vi "Single Beep.vi"(0 "Number of Tones (Def=1)":i32=1) -> ()   [LabVIEW 2020]
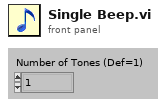
[diagram p1: front panel]
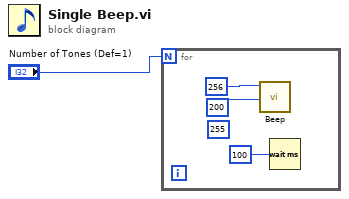
[diagram p0: block diagram]
diagram:
  n1 = for {
    N: "Number of Tones (Def=1)" -> [_]
    (unwired) 255
    n2 = call <vilib>:"Beep.vi"("duration (msec)"=200, "frequency (Hz)"=256) -> ()  [unwired: 10 in]
    n3 = Wait (ms)(milliseconds to wait=100) -> ()  [unwired: 1 out]
  }
